vi "Unflatten From JSON String as Variant Attributes.vi"(8 "error in (no error)":errorcluster, 11 "JSON String":string) -> (0 "error out":errorcluster, 3 "Variant with Attributess":variant)   [LabVIEW 2015, in "JKI JSON Serialization.lvlib"]
doc: "Converts <b>JSON String</b> to <b>Variant</b> with JSON data encoded as Variant Attributes. \n\nIf <b>JSON string</b> is an array, <b>Variant</b> is an array of the appropriate type\n\nIf <b>JSON String</b> is an object, <b>Variant</b> is of null type, with object data encoded as variant attributes.\n\nNo type model is taken as input. If the data types comprising <b>JSON String</b> are known at compile time, use the regular form of <b>Unflatten From JSON String</b>."
uses:
  JKI JSON Serialization.lvlib
  Deserializer/JSON Deserializer/JSON Deserializer.lvclass
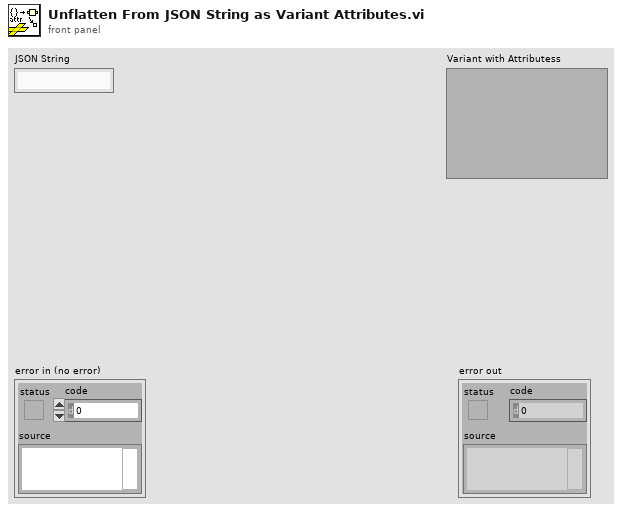
[diagram p1: front panel]
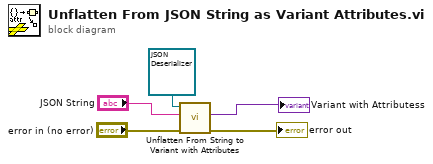
[diagram p0: block diagram]
diagram:
  n1 = call-dynamic "Unflatten From String to Variant with Attributes.vi"("error in (no error)"="error in (no error)", "String"="JSON String", "Deserializer in"=refnum<class "JSON Deserializer.lvclass"> refnum) -> ("error out"=→"error out":errorcluster, "Variant with Attributes"=→"Variant with Attributess":variant)  [unwired: 6 in, 1 out]
